vi "benchmark-massives.vi"() -> ()   [LabVIEW 2022 SP3]
panel:
  out "overall runtime, s":dbl
  out "min time,s":dbl
  out "max time,s":dbl
  in  "No. of runs":i32
  out "Array":dbl[][](array[numeric])
  out "Array size":i32[](array[numeric])
  in  "Array dimensions":dbl[](array[numeric])
  out "Array x10":dbl[][](array[numeric])
  out "Runtime":dbl[](graph)
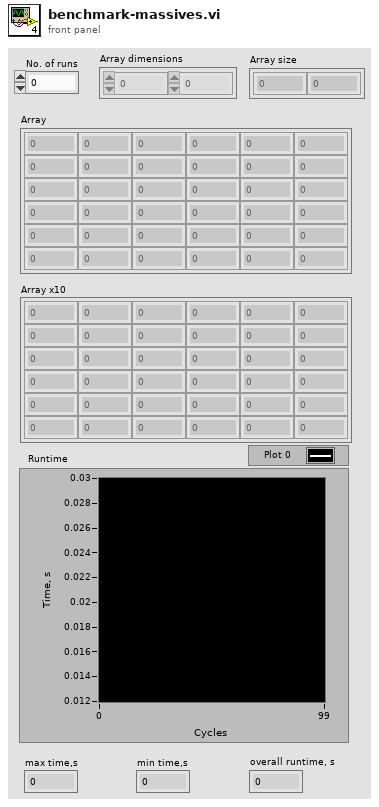
[diagram p1: front panel]
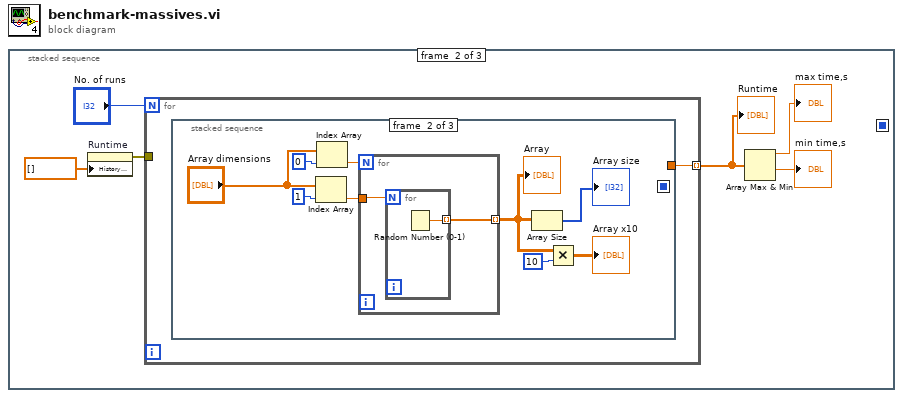
[diagram p0: block diagram]
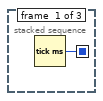
[diagram p2: hidden frame]
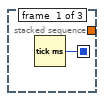
[diagram p3: hidden frame]
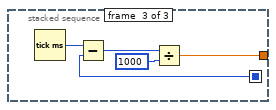
[diagram p4: hidden frame]
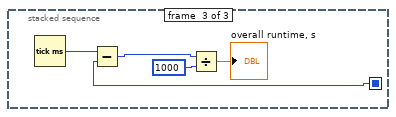
[diagram p5: hidden frame]
diagram:
  n1 = stacked-sequence {
    seq-local: [w1 _ _] -> [_ _ w30]
    frame #0 {
      n2 = Tick Count (ms)() -> (millisecond timer value=w1:u32)
    }
    frame #1 {
      n3 = property on="Runtime" class="WFChart (strict)"("History Data"=dbl[] []) -> (error out=w6:errorcluster)  [unwired: 2 in, 1 out]
      n4 = for {
        N: "No. of runs" -> [_]
        tunnel: w6 -> [_]
        tunnel: [w8] -> w4 mode=indexing
        n5 = stacked-sequence {
          seq-local: [w9 _ _] -> [_ _ w25]
          tunnel: [_ _ w22] -> w8
          frame #0 {
            n6 = Tick Count (ms)() -> (millisecond timer value=w9:u32)
          }
          frame #1 {
            n7 = Index Array(array="Array dimensions", index=1) -> (element=w13:dbl)
            n8 = Index Array(array="Array dimensions", index=0) -> (element=w14:dbl)
            n9 = for {
              N: w14 -> [_]
              tunnel: [w20] -> w12 mode=indexing
              tunnel: w13 -> [w19]
              n10 = for {
                N: w19 -> [_]
                tunnel: [w21] -> w20 mode=indexing
                n11 = Random Number (0-1)() -> (number: 0 to 1=w21:dbl)
              }
            }
            "Array" <- w12
            n12 = Array Size(array=w12) -> (size(s)=→"Array size":i32[])
            n13 = Multiply(x=w12, y=10) -> (x*y=→"Array x10":dbl[][])
          }
          frame #2 {
            n14 = Tick Count (ms)() -> (millisecond timer value=w26:u32)
            n15 = Subtract(x=w26, y=w25) -> (x-y=w24:u32)
            n16 = Divide(x=w24, y=u32 1000) -> (x/y=w22:dbl)
          }
        }
      }
      "Runtime" <- w4
      n17 = Array Max & Min(array=w4) -> (max value=→"max time,s":dbl, min value=→"min time,s":dbl)  [unwired: 2 out]
    }
    frame #2 {
      n18 = Tick Count (ms)() -> (millisecond timer value=w31:u32)
      n19 = Subtract(x=w31, y=w30) -> (x-y=w29:u32)
      n20 = Divide(x=w29, y=u32 1000) -> (x/y=→"overall runtime, s":dbl)
    }
  }
